vi "字符串与U8数组之间转换.vi"() -> ()   [LabVIEW 2022 SP3]
doc: "本VI是为《我和LabVIEW》一书编写的示例。\n关于本书的介绍请参考网页：\nhttp://ruanqizhen.spaces.live.com/blog/cns!5852D4F797C53FB6!4310.entry"
panel:
  out "无符号字节数组 2":u8[](array[numeric]) format="%.0x"
  out "无符号字节数组":u8[](array[numeric])
  out "字符串 2":string
  out "字符串":string
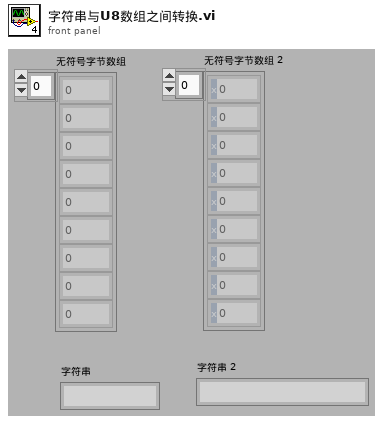
[diagram p1: front panel]
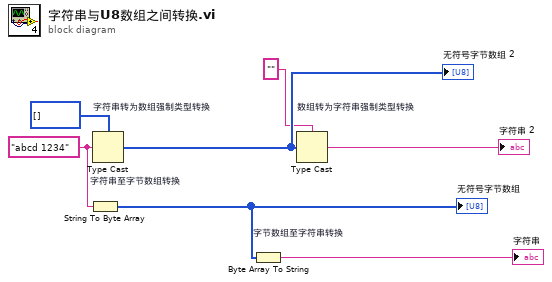
[diagram p0: block diagram]
diagram:
  w5 = "abcd 1234"
  n1 = String To Byte Array "字符串至字节数组转换"(string=w5) -> (unsigned byte array=w6:u8[])
  "无符号字节数组" <- w6
  n2 = Type Cast "字符串转为数组强制类型转换"(type=u8[] [] ("无符号字节数组"), x=w5) -> (*(type *) &x=w3:u8[])
  "无符号字节数组 2" <- w3
  n3 = Byte Array To String "字节数组至字符串转换"(unsigned byte array=w6) -> (string=→"字符串":string)
  n4 = Type Cast "数组转为字符串强制类型转换"(type="" ("类型"), x=w3) -> (*(type *) &x=→"字符串 2":string)
